vi "RIOduino_COM.vi"   [LabVIEW 2014]
types:
  T1 = typedef "WPI_I2CDevRef.ctl" = cluster{"DevStatus":errorcluster, "Controller":T2, "Device Address":u8, "Handle":i32, "I2C Bus":T3}
  T2 = typedef "FPGA_TypedefDigitalModule.ctl" = enum16{"Controller 1"}
  T3 = typedef "i2c_bus.ctl" = enum16{"I2C On-Board", "I2C MXP", "Invalid"}
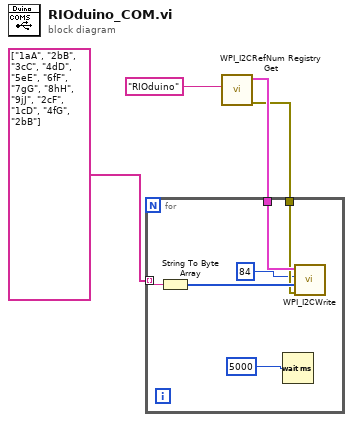
[diagram p0: block diagram]
diagram:
  n1 = call <vilib>:"WPI_I2CRefNum Registry Get.vi"("refnum name"="RIOduino") -> ("error out"=w1:errorcluster, "I2CDevRef"=w2:T1)  [unwired: 9 in]
  n2 = for {
    tunnel: string[] ["1aA", "2bB", "3cC", "4dD", "5eE", "6fF", "7gG", "8hH", "9jJ", "2cF", "1cD", "4fG", "2bB"] -> [w10] mode=indexing
    tunnel: w2 -> [w8]
    tunnel: w1 -> [w7]
    n3 = String To Byte Array(string=w10) -> (unsigned byte array=w9:u8[])
    n4 = Wait (ms)(milliseconds to wait=5000) -> ()  [unwired: 1 out]
    n5 = call <vilib>:"WPI_I2CWrite.vi"("error in (no error)"=w7, "I2CDataToSend"=w9, "I2CRegister"=u8 84, "I2CDevRef"=w8) -> ()  [unwired: 6 in, 2 out]
  }
